vi "SizeCache.vi"(8 "Set":bool, 11 "SizeIn":dbl) -> (3 "SizeOut":dbl)   [LabVIEW 2014]
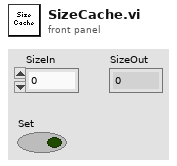
[diagram p1: front panel]
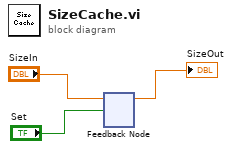
[diagram p0: block diagram]
diagram:
  n1 = feedback-in #1("SizeIn", "Set") -> ()
  n2 = feedback #1() -> (→"SizeOut":dbl)  [unwired: 1 in]
